vi "EXAMPLE APPLICATION.vi"() -> ()   [LabVIEW 2021]
uses:
  <vilib>/Instr/_visa.llb/VISA Configure Serial Port (Instr).vi
panel:
  in  "Slide":dbl(slide) scale=0.0..255.0
  out "Potentiometer: 2":dbl(knob) scale=0.0..255.0
  out "Written?":bool
  out "Data to Send":i32[](array[numeric])
  in  "MED:":dbl
  in  "MIN:":dbl
  in  "MAX:":dbl
  out "(hi.lo)":u16
  out "Potentiometer:":dbl(knob) scale=0.0..1023.0
  in  "Start":bool
  in  "Write?":bool
  out "DBarray":dbl[][](array[numeric])
  in  "DB File":string="cansart_db.h"
  in  "stop":bool
  in  "BaudRate:":u32=115200
  in  "COM:":refnum<visa-resource-name>
  # "Cansart Example Application"
  # "Test Potentiometer by connecting a potentiometer\non the pin referred on your controller example"
  # "Double Click on the 1023 number to change it \nto a higher number depending on what your \nADC resolution"
  # "Engineered and Maintained by:\nGuilherme Candido\nteoriaeletrica@gmail.com"
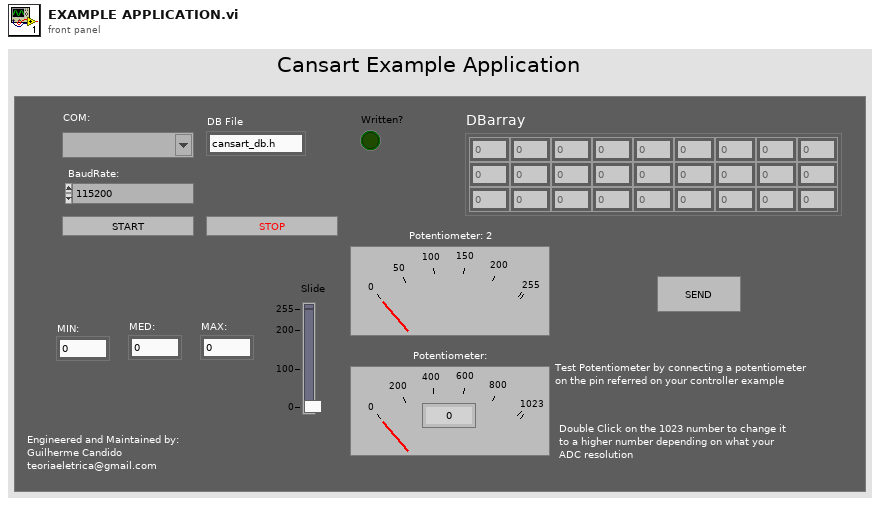
[diagram p1: front panel]
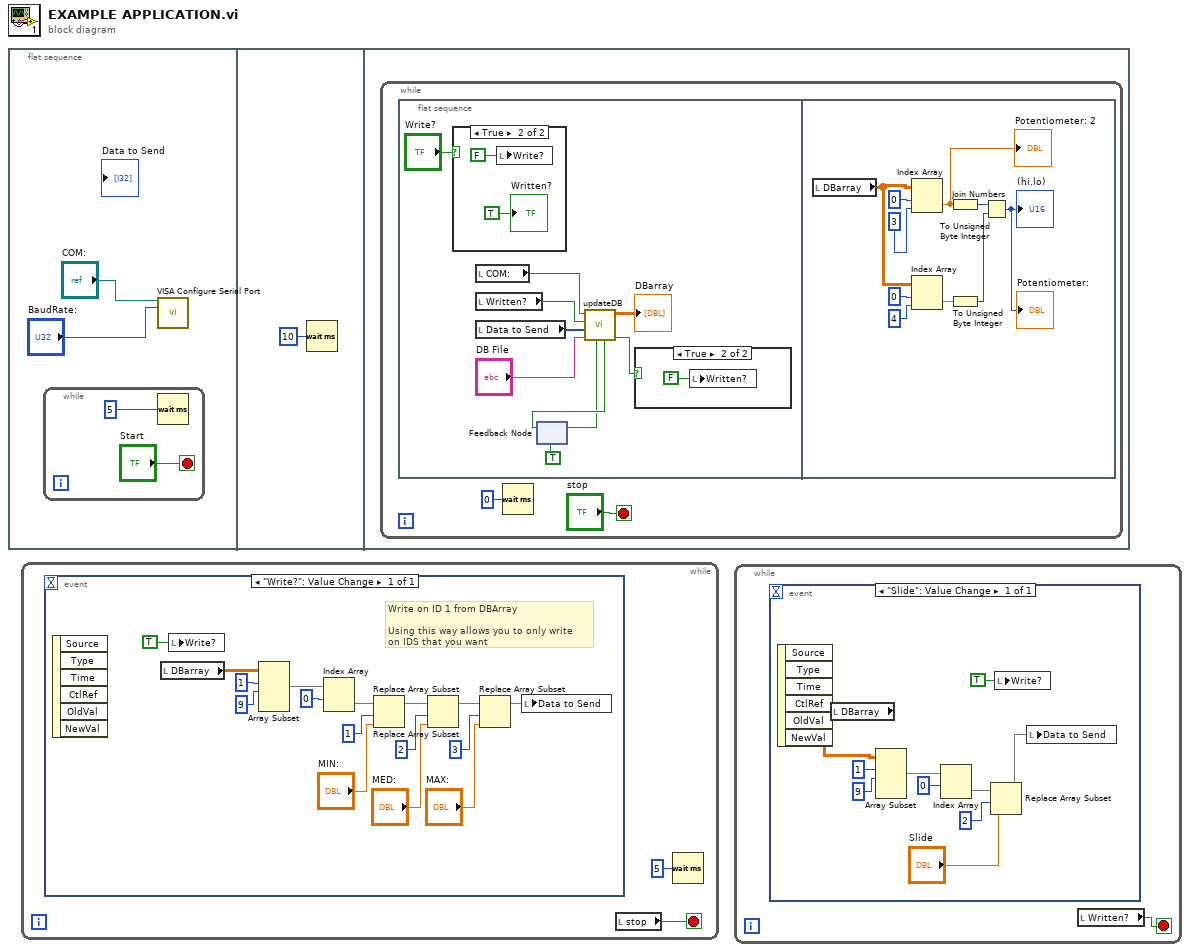
[diagram p0: block diagram]
diagram:
  n1 = flat-sequence {
    frame #0 {
      n2 = while {
        stop <- "Start" stop-if-true
        n3 = Wait (ms)(milliseconds to wait=u32 5) -> ()  [unwired: 1 out]
      }
      n4 = call-poly "VISA Configure Serial Port"("VISA resource name"="COM:", "baud rate (9600)"="BaudRate:") -> ()  [unwired: 12 in, 2 out]
    }
    frame #1 {
      n5 = Wait (ms)(milliseconds to wait=u32 10) -> ()  [unwired: 1 out]
    }
    frame #2 {
      n6 = while {
        stop <- "stop" stop-if-true
        n7 = flat-sequence {
          frame #0 {
            n8 = case shown="True" "Write?" {
              frame False {
              }
              frame True {
                n9 = local write "Write?"(FALSE ("Write?")) -> ()
                "Written?" <- TRUE ("Boolean")
              }
            }
            n10 = local read "COM:"() -> (w17:refnum<visa-resource-name>)
            n11 = local read "Written?"() -> (w8:bool)
            n12 = local read "Data to Send"() -> (w11:i32[])
            n13 = feedback #1(TRUE ("First 2")) -> (w13:bool)
            n14 = call "updateDB.vi"("First"=w13, "DBname"="DB File", "Data Write"=w11, "Write?"=w8, "COM PORT"=w17) -> ("Written!"=w9:bool, "DBarray"=→"DBarray":dbl[][], "First 2"=w14:bool)  [unwired: 4 in]
            n15 = feedback-in #1(w14) -> ()
            n16 = case shown="True" w9 {
              frame False {
              }
              frame True {
                n17 = local write "Written?"(FALSE ("Written?")) -> ()
              }
            }
          }
          frame #1 {
            n18 = local read "DBarray"() -> (w28:dbl[][])
            n19 = Index Array(array=w28, index (row)=0, index (col)=3 ("disabled index (col)")) -> (element=w21:dbl)
            "Potentiometer: 2" <- w21
            n20 = Index Array(array=w28, index (row)=0, index (col)=4 ("disabled index (col)")) -> (element=w24:dbl)
            n21 = To Unsigned Byte Integer(number=w21) -> (unsigned 8bit integer=w25:u8)
            n22 = To Unsigned Byte Integer(number=w24) -> (unsigned 8bit integer=w23:u8)
            n23 = Join Numbers(hi=w25, lo=w23) -> ((hi.lo)=→"(hi.lo)" →"Potentiometer:":u16)
          }
        }
        n24 = Wait (ms)(milliseconds to wait=u32 0) -> ()  [unwired: 1 out]
      }
    }
  }
  n25 = while {
    stop <- w32 stop-if-true
    n26 = event shown="[0] \"Write?\": Value Change" {
      selector: _ -> [_]
      dyn-events: _ -> [_]
      timeout: _ -> [_]
      event "Write?": Value Change {
        # "Write on ID 1 from DBArray\n\nUsing this way allows you to only write\non IDS that you want"
        n27 = event-data() -> ()  [unwired: 1 in, 6 out]
        n28 = local read "DBarray"() -> (w41:dbl[][])
        n29 = local write "Write?"(TRUE ("Write?")) -> ()
        n30 = Array Subset(array=w41, index (row)=1 ("index"), length (row)=9 ("length")) -> (w48:dbl[][])  [unwired: 2 in]
        n31 = Index Array(array=w48, index (row)=0) -> (element=w40:dbl[])  [unwired: 1 in]
        n32 = Replace Array Subset(array=w40, new element="MIN:", index=1) -> (w47:dbl[])
        n33 = Replace Array Subset(array=w47, new element="MED:", index=2) -> (w36:dbl[])
        n34 = Replace Array Subset(array=w36, new element="MAX:", index=3) -> (w33:dbl[])
        n35 = local write "Data to Send"(w33) -> ()
      }
    }
    n36 = local read "stop"() -> (w32:bool)
    n37 = Wait (ms)(milliseconds to wait=u32 5) -> ()  [unwired: 1 out]
  }
  n38 = while {
    stop <- w49 stop-if-true
    n39 = event shown="[0] \"Slide\": Value Change" {
      selector: _ -> [_]
      dyn-events: _ -> [_]
      timeout: _ -> [_]
      event "Slide": Value Change {
        n40 = event-data() -> ()  [unwired: 1 in, 6 out]
        n41 = local read "DBarray"() -> (w53:dbl[][])
        n42 = Array Subset(array=w53, index (row)=1 ("index"), length (row)=9 ("length")) -> (w58:dbl[][])  [unwired: 2 in]
        n43 = Index Array(array=w58, index (row)=0) -> (element=w59:dbl[])  [unwired: 1 in]
        n44 = Replace Array Subset(array=w59, new element="Slide", index=2) -> (w51:dbl[])
        n45 = local write "Write?"(TRUE ("Write?")) -> ()
        n46 = local write "Data to Send"(w51) -> ()
      }
    }
    n47 = local read "Written?"() -> (w49:bool)
  }
